vi "Communication Module.vi"(8 "error in (no error)":errorcluster, 10 "Data Proecss":refnum<queue>, 11 "Queue in":refnum<queue>) -> (0 "error out":errorcluster)   [LabVIEW 2020]
uses:
  Libraries/Message Queue/Message Cluster.ctl
  Controls/Comm Data.ctl
  Libraries/Message Queue/Enqueue Message (Single).vi
  <vilib>/Utility/error.llb/Error Cluster From Error Code.vi
  <vilib>/ErrorRing/Error Ring.xnode
  Libraries/Message Queue/Message Queue.lvlib
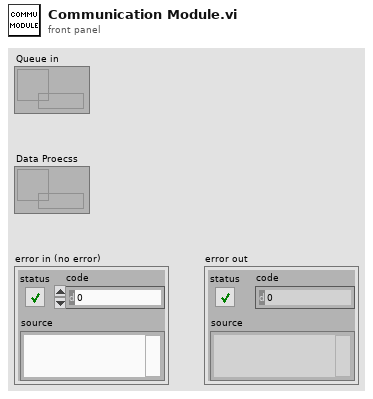
[diagram p1: front panel]
types:
  T1 = typedef "Comm Data.ctl" = cluster{"VISA":refnum<visa-resource-name>}
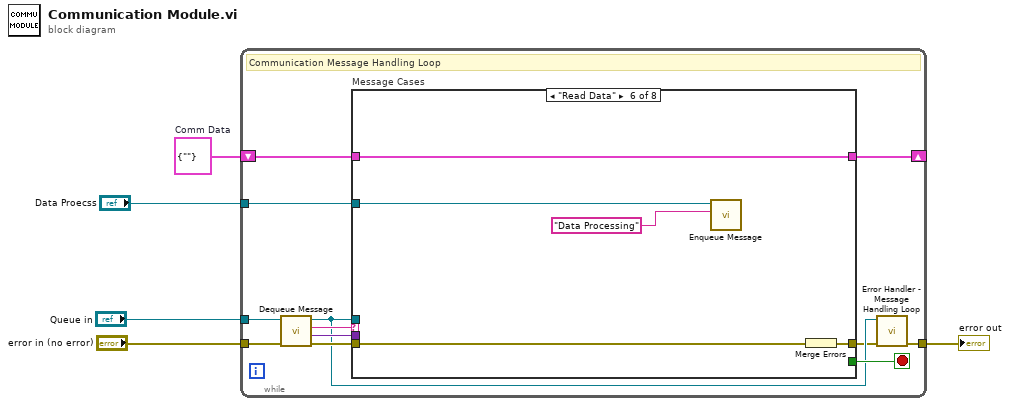
[diagram p0: block diagram]
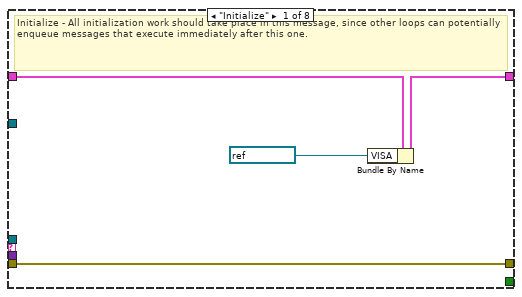
[diagram p2: hidden frame]
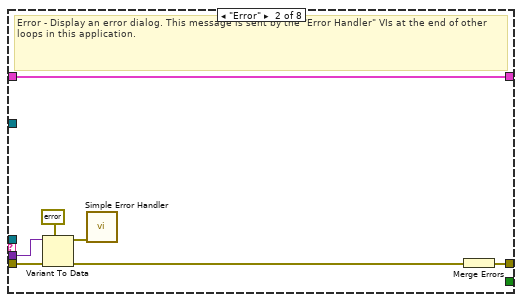
[diagram p3: hidden frame]
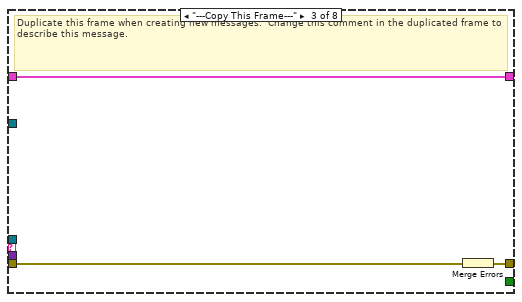
[diagram p4: hidden frame]
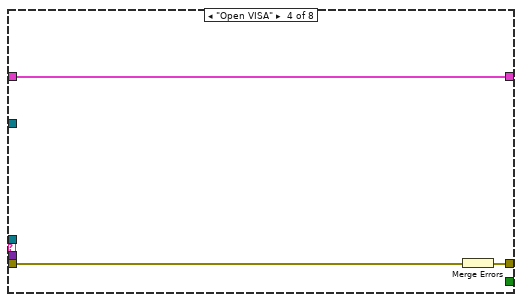
[diagram p5: hidden frame]
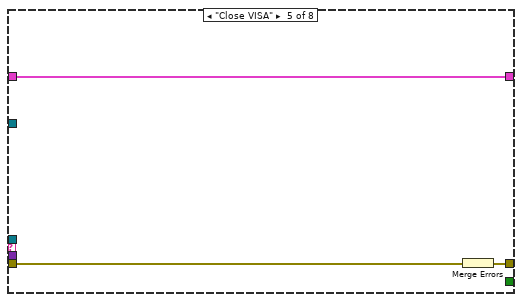
[diagram p6: hidden frame]
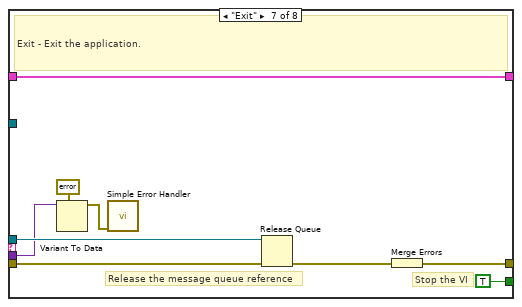
[diagram p7: hidden frame]
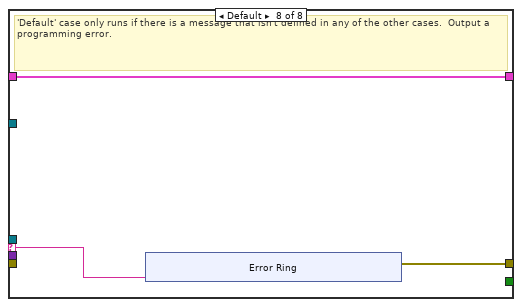
[diagram p8: hidden frame]
diagram:
  w4 = T1 {"VISA"=""}  # Comm Data
  n1 = while {
    tunnel: "Queue in" -> [w10]
    shift-right: [w16] -> _
    shift-left: w4 -> [w17]
    tunnel: "error in (no error)" -> [w14]
    tunnel: [w8] -> w3
    tunnel: "Data Proecss" -> [w6]
    stop <- w15 stop-if-true
    # "Communication Message Handling Loop"
    n2 = call "Dequeue Message.vi"("error in (no error)"=w14, "Message Queue"=w10) -> ("error out"=w13:errorcluster, "Message Data"=w11:variant, "Message"=w12:string, "dup Message Queue"=w9:refnum<queue>)  [unwired: 6 in]
    n3 = case "Message Cases" shown="\"Read Data\"" w12 {
      selector: w12 -> [_ _ _ _ _ _ _ w52]
      tunnel: w9 -> [_ _ _ _ _ _ w51 _]
      tunnel: w13 -> [w21 w28 w31 w34 w37 w42 w47 _]
      tunnel: [w21 w22 w29 w32 w35 w40 w48 w53] -> w7
      tunnel: w17 -> [w20 w27 w30 w33 w36 w41 w43 w54]
      tunnel: [w19 w27 w30 w33 w36 w41 w43 w54] -> w16
      tunnel: [_ _ _ _ _ _ TRUE _] -> w15
      tunnel: w11 -> [_ w26 _ _ _ _ w44 _]
      tunnel: w6 -> [_ _ _ _ _ w39 _ _]
      frame "Initialize" {
        # "Initialize - All initialization work should take place in this message, since other loops can potentially enqueue messages that execute immediately after this one."
        n4 = Bundle By Name(cluster=w20, "VISA"=refnum<visa-resource-name> "COM50") -> (w19:T1)
      }
      frame "Error" {
        # "Error - Display an error dialog. This message is sent by the \"Error Handler\" VIs at the end of other loops in this application."
        n5 = Variant To Data(error in=w28, type=errorcluster {"status"=FALSE, "code"=0, "source"=""} ("error constant"), Variant=w26) -> (data=w24:errorcluster, error out=w23:errorcluster)
        n6 = call <vilib>:"Simple Error Handler.vi"("error in (no error)"=w24) -> ()  [unwired: 4 in, 5 out]
        n7 = Merge Errors(w23) -> (w22:errorcluster)
      }
      frame "---Copy This Frame---" {
        # "Duplicate this frame when creating new messages.  Change this comment in the duplicated frame to describe this message."
        n8 = Merge Errors(w31) -> (w29:errorcluster)
      }
      frame "Open VISA" {
        n9 = Merge Errors(w34) -> (w32:errorcluster)
      }
      frame "Close VISA" {
        n10 = Merge Errors(w37) -> (w35:errorcluster)
      }
      frame "Read Data" {
        n11 = call-poly "Enqueue Message.vi"("Message"="Data Processing", "Message Queue"=w39) -> ()  [unwired: 8 in, 2 out]
        n12 = Merge Errors(w42) -> (w40:errorcluster)
      }
      frame "Exit" {
        # "Stop the VI"
        # "Release the message queue reference"
        # "Exit - Exit the application."
        n13 = Variant To Data(type=errorcluster {"status"=FALSE, "code"=0, "source"=""} ("error constant"), Variant=w44) -> (data=w45:errorcluster)  [unwired: 1 in, 1 out]
        n14 = call <vilib>:"Simple Error Handler.vi"("error in (no error)"=w45) -> ()  [unwired: 4 in, 5 out]
        n15 = Release Queue(queue=w51, error in (no error)=w47) -> (error out=w49:errorcluster)  [unwired: 1 in, 2 out]
        n16 = Merge Errors(w49) -> (w48:errorcluster)
      }
      frame Default {
        # "'Default' case only runs if there is a message that isn't defined in any of the other cases.  Output a programming error."
        n17 = xnode "Error Ring"("parameter 0"=w52) -> ("error out"=w53:errorcluster)
      }
    }
    n18 = call "Error Handler - Message Handling Loop.vi"("error in (no error)"=w7, "Message Queue"=w9) -> ("dup error in"=w8:errorcluster)  [unwired: 8 in, 1 out]
  }
  "error out" <- w3
